vi "Default Reversed By Name.vi"(10 "This is Array?":bool, 11 "RelationPanel in":refnum<class "RelationPanel.lvclass">) -> (2 "Default Reversed By":string)   [LabVIEW 2020, in "Conditum-Tools.lvlib" / "RelationPanel.lvclass"]
uses:
  RelationPanel.lvclass
  RelationPanel.lvclass/RelationPanel.ctl
  Conditum-Tools.lvlib
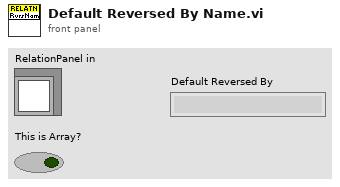
[diagram p1: front panel]
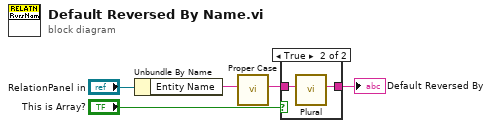
[diagram p0: block diagram]
diagram:
  n1 = Unbundle By Name("RelationPanel in") -> ("Entity Name"=w3:string)
  n2 = call "Proper Case.vi"("String in"=w3) -> ("Proper Cased"=w2:string)  [unwired: 10 in]
  n3 = case shown="True" "This is Array?" {
    tunnel: w2 -> [w6 w8]
    tunnel: [w6 w7] -> w1
    frame False {
    }
    frame True {
      n4 = call "Plural.vi"("String"=w8) -> ("Plural"=w7:string)  [unwired: 10 in]
    }
  }
  "Default Reversed By" <- w1
